vi "ADCdata_to_mV.vi"(10 "ADC data":u16, 11 "ADC PGA":u8) -> (3 "mV/lux ouptut":dbl)   [LabVIEW 2013]
panel:
  out "Numeric 2":dbl
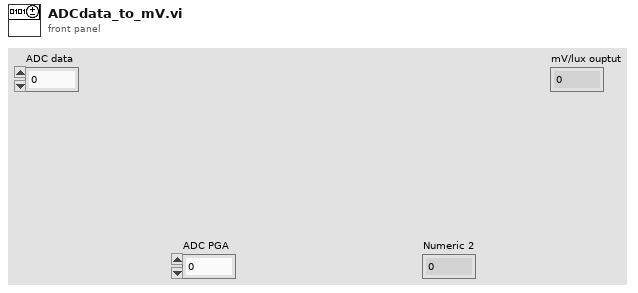
[diagram p1: front panel]
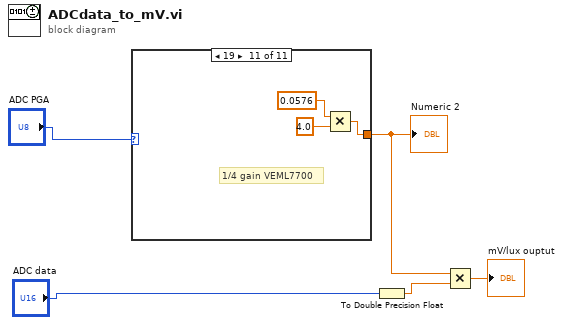
[diagram p0: block diagram]
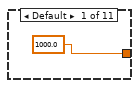
[diagram p2: hidden frame]
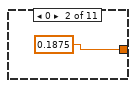
[diagram p3: hidden frame]
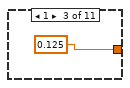
[diagram p4: hidden frame]
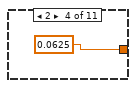
[diagram p5: hidden frame]
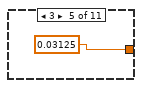
[diagram p6: hidden frame]
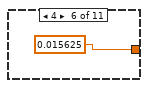
[diagram p7: hidden frame]
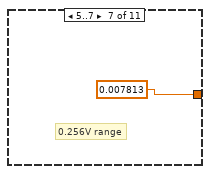
[diagram p8: hidden frame]
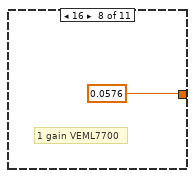
[diagram p9: hidden frame]
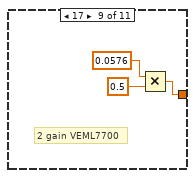
[diagram p10: hidden frame]
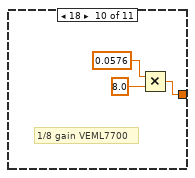
[diagram p11: hidden frame]
diagram:
  n1 = case shown="19" "ADC PGA" {
    tunnel: [1000.0 ("Numeric 2") 0.1875 ("Numeric 2") 0.125 ("Numeric 2") 0.0625 ("Numeric 2") 0.03125 ("Numeric 2") 0.015625 ("Numeric 2") 0.007813 ("Numeric 2") 0.0576 ("Numeric 2") w16 w19 w22] -> w4
    frame Default {
    }
    frame 0 {
    }
    frame 1 {
    }
    frame 2 {
    }
    frame 3 {
    }
    frame 4 {
    }
    frame 5..7 {
      # "0.256V range"
    }
    frame 16 {
      # "1 gain VEML7700"
    }
    frame 17 {
      # "2 gain VEML7700"
      n2 = Multiply(x=0.0576 ("Numeric 2"), y=0.5) -> (x*y=w16:dbl)
    }
    frame 18 {
      # "1/8 gain VEML7700"
      n3 = Multiply(x=0.0576 ("Numeric 2"), y=8.0) -> (x*y=w19:dbl)
    }
    frame 19 {
      # "1/4 gain VEML7700"
      n4 = Multiply(x=0.0576 ("Numeric 2"), y=4.0) -> (x*y=w22:dbl)
    }
  }
  "Numeric 2" <- w4
  n5 = To Double Precision Float(number="ADC data") -> (double precision float=w3:dbl)
  n6 = Multiply(x=w4, y=w3) -> (x*y=→"mV/lux ouptut":dbl)
